vi "Close.vi"(8 "error in (no error)":errorcluster, 11 "Inst.RP100 in":refnum<class "Inst.RP100.lvclass">) -> (0 "error out":errorcluster, 3 "Inst.RP100 out":refnum<class "Inst.RP100.lvclass">)   [LabVIEW 2019, in "Inst.RP100.lvlib" / "Inst.RP100.lvclass"]
uses:
  Inst.RP100.lvclass
  C:/Program Files (x86)/National Instruments/LabVIEW 2019/user.lib/LevyLab/Instrument Framework/Instrument/Instrument.lvclass
  <userlib>/LevyLab/Instrument Framework/Instrument Types/Strain/Instrument.Strain.lvclass
  <userlib>/LevyLab/Instrument Framework/Instrument/Instrument.lvclass
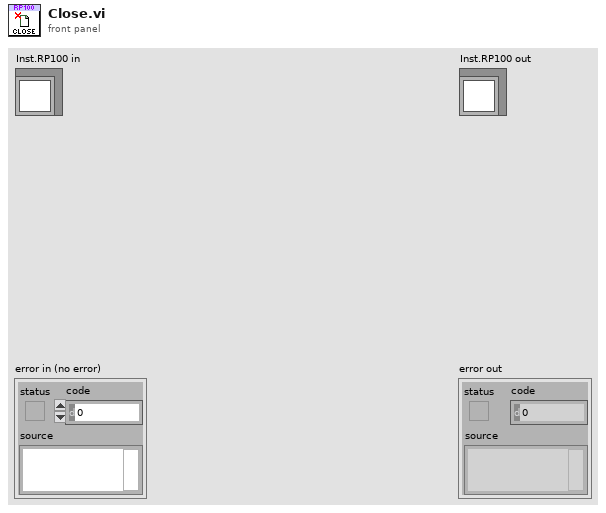
[diagram p1: front panel]
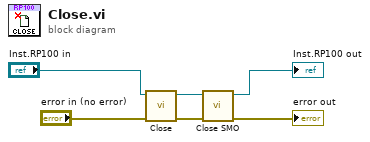
[diagram p0: block diagram]
diagram:
  n1 = call-parent "Close.vi"("error in (no error)"="error in (no error)", "Instrument in"="Inst.RP100 in") -> ("error out"=w4:errorcluster, "Instrument out"=w3:refnum<class "Inst.RP100.lvclass">)  [unwired: 8 in]
  n2 = call <userlib>:"Close SMO.vi"("error in (no error)"=w4, "Instrument in"=w3) -> ("error out"=→"error out":errorcluster, "Instrument out"=→"Inst.RP100 out":refnum<class "Inst.RP100.lvclass">)  [unwired: 8 in]
